vi "Parsed XML To System Definition.vi"(8 "error in":errorcluster, 9 "path to XML document":path caption="path to parameters xml", 10 "ports":T2[](array[typedef]), 11 "custom device ref":T1 format="%.0x") -> (0 "error out":errorcluster, 3 "custom device ref out":T1 format="%.0x")   [LabVIEW 2020, in "Ballard ARINC 429 Scripting.lvlib"]
uses:
  Ballard ARINC 429 Scripting.lvlib
  <vilib>/NI VeriStand/Custom Device API/Custom Device Item Ref.ctl
  Shared/VS Channels Definition for All Labels on Hardware Channel.ctl
  Shared/VS Channels Definition for Label.ctl
  Shared/VS Channel Definition for Parameter.ctl
  Shared/Direction.ctl
  Shared/Parameter Definition.ctl
  Encoding and Decoding/Encoding.ctl
  Shared/Transfer Type.ctl
  <vilib>/NI VeriStand/Custom Device API/Custom Device API.lvlib
  Encoding and Decoding/Encoding and Decoding.lvlib
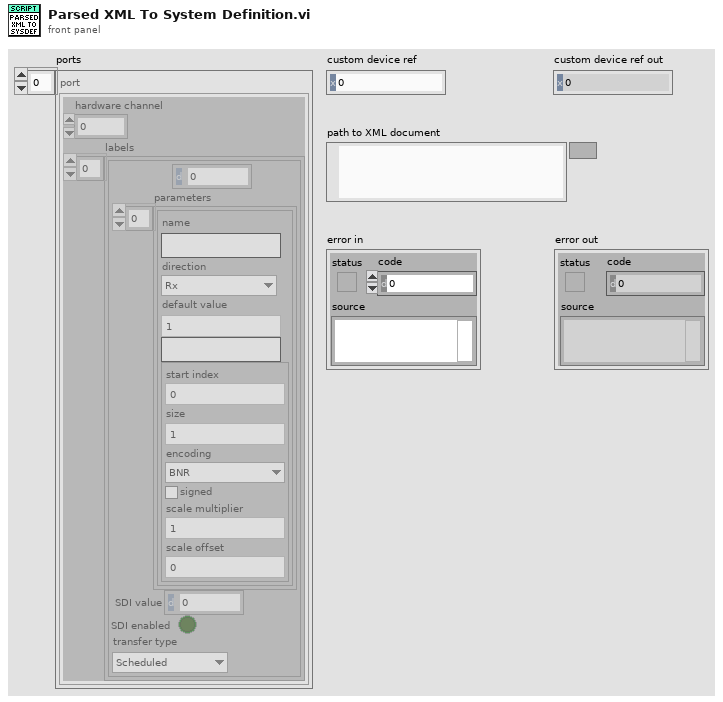
[diagram p1: front panel]
types:
  T1 = typedef "Custom Device API.lvlib/Custom Device Item Ref.ctl" = u64
  T2 = typedef "VS Channels Definition for All Labels on Hardware Channel.ctl" = cluster{"hardware channel":i32, "labels":T3[]}
  T3 = typedef "VS Channels Definition for Label.ctl" = cluster{"label (Dec)":u32, "parameters":T4[], "SDI value":u8, "SDI enabled":bool, "transfer type":T8}
  T4 = typedef "VS Channel Definition for Parameter.ctl" = cluster{"name":string, "direction":T5, "default value":dbl, "unit":string, "Parameter":T6}
  T5 = typedef "Direction.ctl" = enum16{"Rx", "Tx"}
  T6 = typedef "Parameter Definition.ctl" = cluster{"start index":i32, "size":i32, "encoding":T7, "signed":bool, "scale multiplier":dbl, "scale offset":dbl}
  T7 = typedef "Encoding and Decoding.lvlib/Encoding.ctl" = enum16{"BNR", "BCD", "Discrete"}
  T8 = typedef "Transfer Type.ctl" = enum16{"Scheduled", "Acyclic", "Block", "Strobe"}
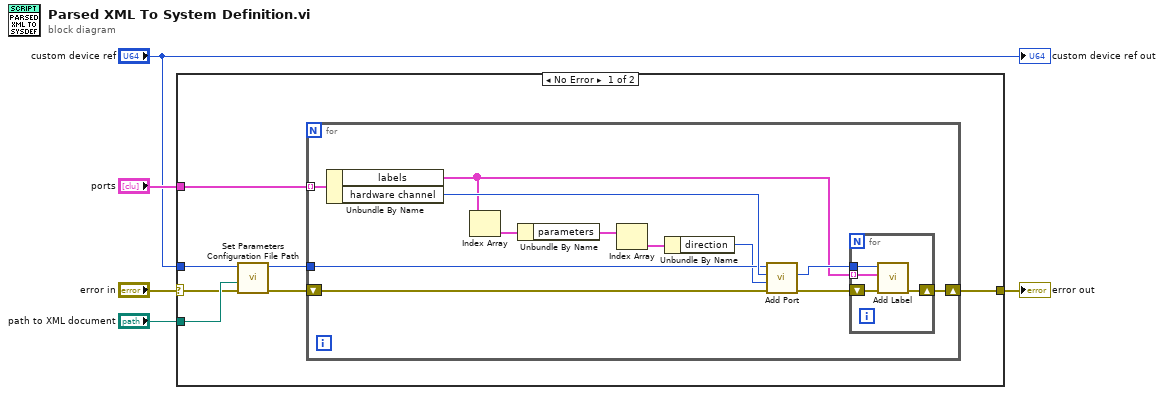
[diagram p0: block diagram]
diagram:
  n1 = case shown="No Error" "error in" {
    selector: "error in" -> [w8 w29]
    tunnel: "custom device ref" -> [w7 _]
    tunnel: [w12 w29] -> w5
    tunnel: "ports" -> [w11 _]
    tunnel: "path to XML document" -> [w9 _]
    frame No Error {
      n2 = call "Set Parameters Configuration File Path.vi"("error in"=w8, "Path"=w9, "Custom device Ref"=w7) -> ("error out"=w10:errorcluster, "Custom device Ref out"=w6:T1)  [unwired: 7 in]
      n3 = for {
        shift-right: [w21] -> w12
        shift-left: w10 -> [w18]
        tunnel: w6 -> [w19]
        tunnel: w11 -> [w24] mode=indexing
        n4 = Unbundle By Name(w24) -> ("labels"=w17:T3[], "hardware channel"=w20:i32)
        n5 = Index Array(array=w17) -> (element=w16:T3)  [unwired: 1 in]
        n6 = Unbundle By Name(w16) -> ("parameters"=w15:T4[])
        n7 = Index Array(array=w15) -> (element=w14:T4)  [unwired: 1 in]
        n8 = Unbundle By Name(w14) -> ("direction"=w13:T5)
        n9 = call "Add Port.vi"("error in"=w18, "direction"=w13, "port number"=w20, "custom device ref"=w19) -> ("error out"=w23:errorcluster, "port ref out"=w22:T1)  [unwired: 5 in, 1 out]
        n10 = for {
          tunnel: w22 -> [w27]
          tunnel: w17 -> [w26] mode=indexing
          shift-right: [w25] -> w21
          shift-left: w23 -> [w28]
          n11 = call "Add Label.vi"("error in"=w28, "label"=w26, "port ref"=w27) -> ("error out"=w25:errorcluster)  [unwired: 7 in, 1 out]
        }
      }
    }
    frame Error {
    }
  }
  "error out" <- w5
  "custom device ref out" <- "custom device ref"
